vi "Test_AWG_5421_Standalone_SubVIs.vi"(8 "error in (no error)":errorcluster, 10 "AWG 5421 Inputs":T3={"Resource Name"="AWG_5421", "Trigger Type"=2, "Sample Rate"=10000000.0, "Trigger Source"="PFI0"} {"Sample Rate" format="%.2p"; "Trigger Type" items=["None", "Software Edge", "Digital Edge", "Digital Level"]}, 11 "Use Software Trigger":bool=TRUE) -> (0 "error out":errorcluster)   [LabVIEW 2015]
doc: "This VI inits a waveform generation session for AWG-5421. This is a basic example that shows how to setup the board in order to generate waveforms according to a script. \nBy default this configuration uses one channel CH0, and one script trigger ScriptTrigger0. The ScriptTrigger0 is waiting for an external trigger : i.e. a digital Edge on pin PFI 0 by default.\n\nThere are various options for the script to be used. Consult the Script control help for more information on configuring the example for specific scripts."
uses:
  controls/AWG_5421_Inputs.ctl
  <instrlib>/niFgen/niFgen.llb/niFgen_ctl Trigger Source Values (Ring).ctl
  controls/SOFTWARE_Inputs.ctl
panel:
  out "FIFO used":i64
  out "Number of Wfms":i32
  in  "SOFTWARE Inputs":T1={"Application Directory"=path "D:/S.O.F.T.S/LABVIEW/PIL", "Resources Path"=path "D:/S.O.F.T.S/LABVIEW/PIL/resources", "Data Path"=path "D:/PIRENEA/DATA", "XML Path"=path "D:/PIRENEA/DATA", "XML File Filter"="*.xml", "Excit Scripts Path"=path "D:/PIRENEA/EXCIT_SCRIPTS", "Excit Scripts File Filter"="*.txt", "Excit Waveforms Path"=path "D:/PIRENEA/EXCIT_WFMS", "Excit Waveforms File Filter"="*.bin", "Timing Scripts Path"=path "D:/PIRENEA/TIMING_SCRIPTS", "Timing Scripts File Filter"="*.txt", "Timing Waveforms Path"=path "D:/PIRENEA/TIMING_WFMS", "Timing Waveforms File Filter"="*.bin", "Trapping Waveforms Path"=path "D:/PIRENEA/TRAPPING_WFMS", "Trapping Waveforms File Filter"="*.bin"}
  in  "Sample Rate":dbl=20.0 format="%#_13g"
  in  "EXCIT Inputs":T2={"Number of Excitations"=1, "Script text"="script myScript0\n    wait until scriptTrigger0\n    Generate Swift150to550a70dur1200fs20\n    wait until scriptTrigger0\n    Generate Swift150to550a70dur1200fs20\nend script", "Table of Waveforms"=["Swift150to550a70dur1200fs20", "Swift150to550a70dur1200fs20"]} {"Number of Excitations" min=1 max=10}
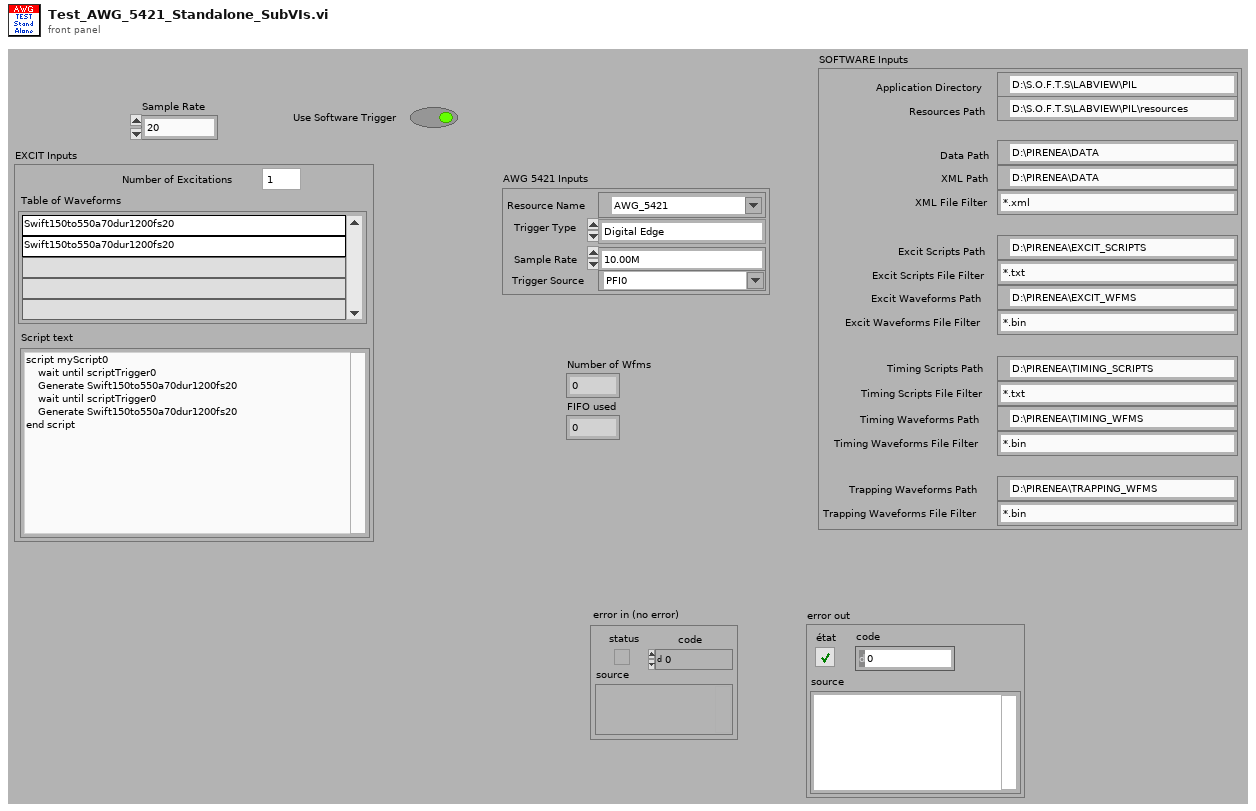
[diagram p1: front panel]
types:
  T1 = typedef "SOFTWARE_Inputs.ctl" = cluster{"Application Directory":path, "Resources Path":path, "Data Path":path, "XML Path":path, "XML File Filter":string, "Excit Scripts Path":path, "Excit Scripts File Filter":string, "Excit Waveforms Path":path, "Excit Waveforms File Filter":string, "Timing Scripts Path":path, "Timing Scripts File Filter":string, "Timing Waveforms Path":path, "Timing Waveforms File Filter":string, "Trapping Waveforms Path":path, "Trapping Waveforms File Filter":string}
  T2 = cluster{"Number of Excitations":i32, "Script text":string, "Table of Waveforms":string[]}
  T3 = typedef "AWG_5421_Inputs.ctl" = cluster{"Resource Name":refnum<k15>, "Trigger Type":u16, "Sample Rate":dbl, "Trigger Source":T4}
  T4 = typedef "niFgen_ctl Trigger Source Values (Ring).ctl" = string
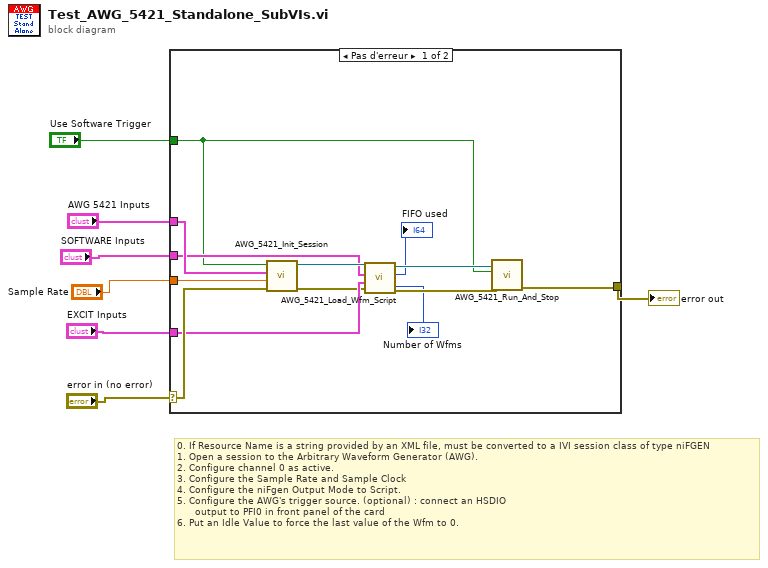
[diagram p0: block diagram]
diagram:
  # "0. If Resource Name is a string provided by an XML file, must be converted to a IVI session class of type niFGEN\n1. Open a session to the Arbitrary Waveform Generator (AWG).\n2. Configure channel 0 as active. \n3. Configure the Sample Rate and Sample Clock\n4. Configure the niFgen Output Mode to Script.\n5. Configure the AWG's trigger source. (optional) : connect an HSDIO\n      output to PFI0 in front panel of the card \n6. Put an Idle Value to force the last value of the Wfm to 0."
  n1 = case shown="Pas d'erreur" "error in (no error)" {
    selector: "error in (no error)" -> [w18 w21]
    tunnel: [w10 w21] -> w7
    tunnel: "AWG 5421 Inputs" -> [w20 _]
    tunnel: "Use Software Trigger" -> [w12 _]
    tunnel: "Sample Rate" -> [w19 _]
    tunnel: "EXCIT Inputs" -> [w16 _]
    tunnel: "SOFTWARE Inputs" -> [w14 _]
    frame No Error {
      n2 = call "AWG_5421_Init_Session.vi"("error in (no error)"=w18, "Sample Rate"=w19, "AWG 5421 Inputs"=w20, "Use Software Trigger"=w12) -> ("error out"=w15:errorcluster, "Instrument handle out"=w17:refnum<k15>)  [unwired: 6 in]
      n3 = call "AWG_5421_Load_Wfm_Script.vi"("error  in"=w15, "EXCIT Inputs"=w16, "SOFTWARE Inputs"=w14, "instrument handle in"=w17) -> ("error out"=w11:errorcluster, "FIFO used"=→"FIFO used":i64, "instrument handle out"=w13:refnum<k15>, "Number of Wfms"=→"Number of Wfms":i32)  [unwired: 3 in, 1 out]
      n4 = call "AWG_5421_Run_And_Stop.vi"("error  in"=w11, "Use Software trigger"=w12, "instrument handle in"=w13) -> ("error out"=w10:errorcluster)  [unwired: 8 in]
    }
    frame Error {
    }
  }
  "error out" <- w7
